vi "lecture2-InitializeArray.vi"() -> ()   [LabVIEW 2014]
panel:
  out "size(s)":i32[](array[numeric])
  in  "Array":bool[][](array[boolean])
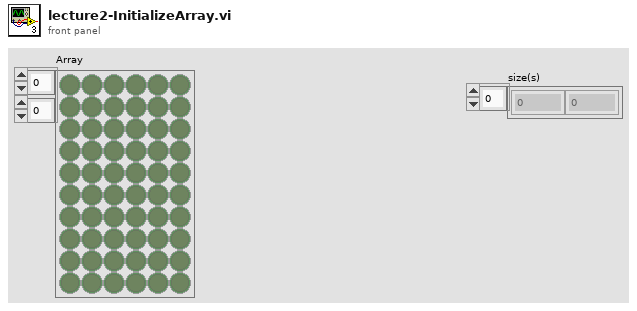
[diagram p1: front panel]
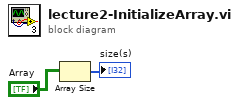
[diagram p0: block diagram]
diagram:
  n1 = Array Size(array="Array") -> (size(s)=→"size(s)":i32[])
